vi "Copy Channel Information.vi"(8 "error in (no error)":errorcluster, 10 "new tdms file":refnum<k34>, 11 "original tdms file":refnum<k34>) -> (0 "error out":errorcluster, 3 "dup original tdms file":refnum<k34>)   [LabVIEW 2023]
doc: "Get all the meta information from the original file and dump them to the new file with TDMS Set Channel Information."
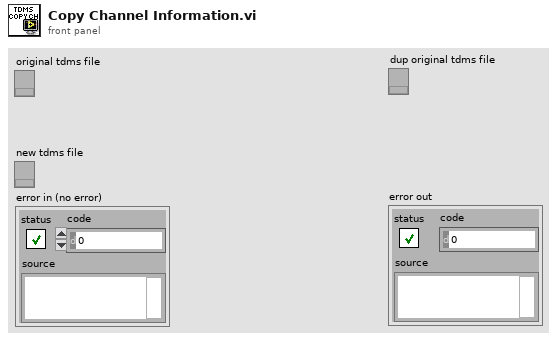
[diagram p1: front panel]
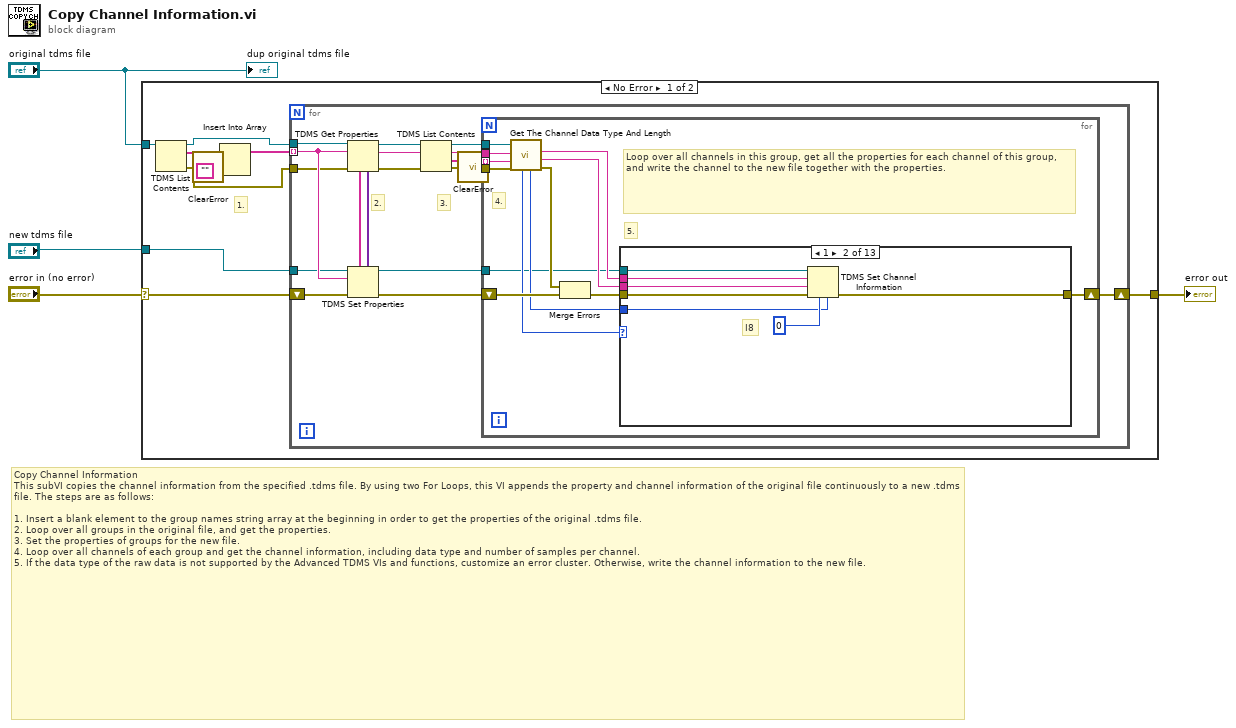
[diagram p0: block diagram]
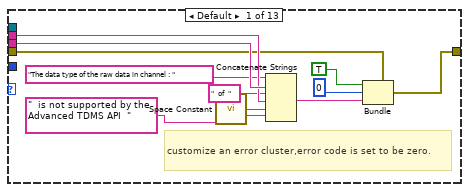
[diagram p2: hidden frame]
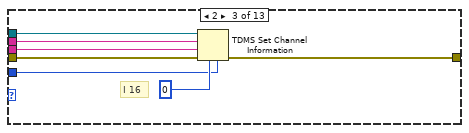
[diagram p3: hidden frame]
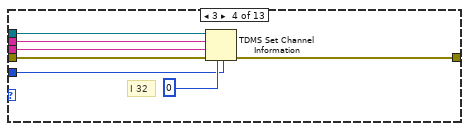
[diagram p4: hidden frame]
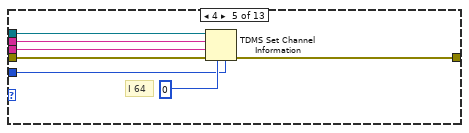
[diagram p5: hidden frame]
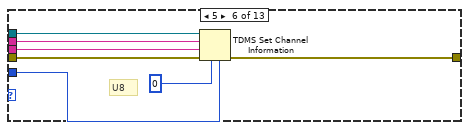
[diagram p6: hidden frame]
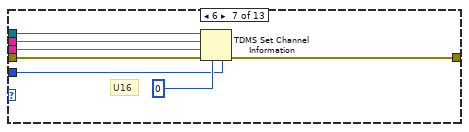
[diagram p7: hidden frame]
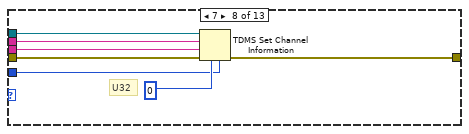
[diagram p8: hidden frame]
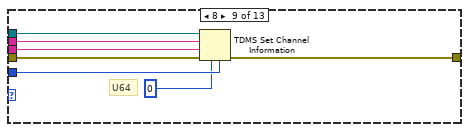
[diagram p9: hidden frame]
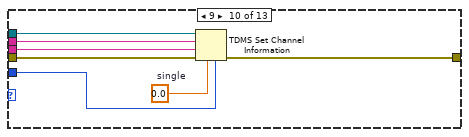
[diagram p10: hidden frame]
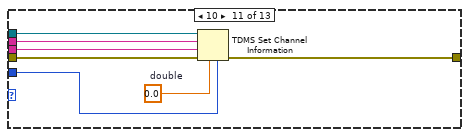
[diagram p11: hidden frame]
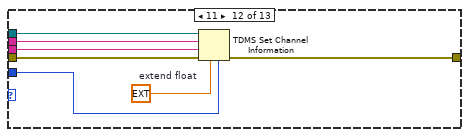
[diagram p12: hidden frame]
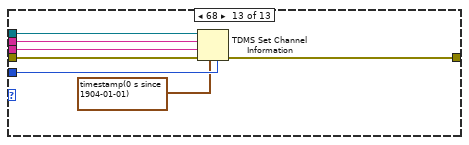
[diagram p13: hidden frame]
diagram:
  # "Copy Channel Information\nThis subVI copies the channel information from the specified .tdms file. By using two For Loops, this VI appends the property and channel information of the original file continuously to a new .tdms file. The steps are as follows:\n\n1. Insert a blank element to the group names string array at the beginning in order to get the properties of the original .tdms file.\n2. Loop over all groups in the original file, and get the properties.\n3. Set the properties of groups for the new file.\n4. Loop over all channels of each group and get the channel information, including data type and number of samples per channel.\n5. If the data type of the raw data is not supported by the Advanced TDMS VIs and functions, customize an error cluster. Otherwise, write the channel information to the new file."
  n1 = case shown="No Error" "error in (no error)" {
    selector: "error in (no error)" -> [w8 w141]
    tunnel: "new tdms file" -> [w6 _]
    tunnel: [w14 w141] -> w3
    tunnel: "original tdms file" -> [w11 _]
    frame No Error {
      # "1."
      n2 = TDMS List Contents(7:w11) -> (0:w5:errorcluster, 2:w9:string[], 3:w10:refnum<k34>)  [unwired: 2 in, 1 out]
      n3 = call <vilib>:"ClearError.vi"("error in (no error)"=w5) -> ("error out"=w7:errorcluster)
      n4 = Insert Into Array(array=w9, new element="" ("new element/subarray")) -> (w12:string[])  [unwired: 1 in]
      n5 = for {
        tunnel: w12 -> [w20] mode=indexing
        shift-right: [w29] -> w14
        shift-left: w8 -> [w18]
        tunnel: w7 -> [w19]
        tunnel: w10 -> [w30]
        tunnel: w6 -> [w17]
        # "3."
        # "2."
        n6 = TDMS Get Properties(8:w19, 10:w20, 11:w30) -> (0:w23:errorcluster, 2:w27:string, 3:w28:refnum<k34>, 4:w31:variant[], 6:w32:string[])  [unwired: 3 in, 1 out]
        n7 = TDMS Set Properties(5:w31, 7:w32, 8:w18, 10:w20, 11:w17) -> (0:w21:errorcluster, 3:w16:refnum<k34>)  [unwired: 1 in, 2 out]
        n8 = TDMS List Contents(4:w23, 6:w27, 7:w28) -> (0:w15:errorcluster, 1:w24:string[], 2:w25:string, 3:w26:refnum<k34>)
        n9 = call <vilib>:"ClearError.vi"("error in (no error)"=w15) -> ("error out"=w22:errorcluster)
        n10 = for {
          shift-right: [w45] -> w29
          shift-left: w21 -> [w38]
          tunnel: w25 -> [w41]
          tunnel: w24 -> [w40] mode=indexing
          tunnel: w22 -> [w39]
          tunnel: w26 -> [w42]
          tunnel: w16 -> [w33]
          # "5."
          # "4."
          # "Loop over all channels in this group, get all the properties for each channel of this group, and write the channel to the new file together with the properties."
          n11 = call "Get The Channel Data Type And Length.vi"("error in (no error)"=w39, "channel name"=w40, "group name"=w41, "tdms file"=w42) -> ("error out"=w44:errorcluster, "dup channel name"=w34:string, "dup group name"=w35:string, "channel length"=w37:i32, "data type"=w36:i32)  [unwired: 2 in, 1 out]
          n12 = Merge Errors(w44, w38) -> (w43:errorcluster)
          n13 = case shown="1" w36 {
            tunnel: w37 -> [_ w62 w68 w76 w83 w85 w96 w103 w112 w113 w120 w127 w139]
            tunnel: w33 -> [_ w61 w70 w75 w82 w91 w98 w105 w110 w118 w125 w133 w140]
            tunnel: w35 -> [w54 w60 w66 w74 w81 w90 w95 w102 w109 w117 w123 w131 w137]
            tunnel: w34 -> [w56 w59 w67 w73 w80 w89 w94 w101 w108 w116 w124 w132 w136]
            tunnel: w43 -> [w50 w58 w65 w72 w79 w87 w93 w100 w107 w115 w122 w130 w135]
            tunnel: [w46 w57 w64 w71 w78 w86 w92 w99 w106 w114 w121 w129 w134] -> w45
            frame Default {
              # "customize an error cluster,error code is set to be zero."
              n14 = call <vilib>:"Space Constant.vi"() -> ("String"=w55:string)
              n15 = Concatenate Strings("The data type of the raw data in channel : " ("message"), w56, "  of  ", w54, w55, "  is not supported by the Advanced TDMS API  " ("message")) -> (w49:string)
              n16 = Bundle(cluster=w50, "status"=TRUE, "code"=0, "source"=w49) -> (w46:errorcluster)
            }
            frame 1 {
              # "I8"
              n17 = TDMS Set Channel Information(4:w62, 6:i8 0, 8:w58, 9:w59, 10:w60, 11:w61) -> (0:w57:errorcluster)  [unwired: 1 in, 1 out]
            }
            frame 2 {
              # "I 16"
              n18 = TDMS Set Channel Information(4:w68, 6:i16 0, 8:w65, 9:w67, 10:w66, 11:w70) -> (0:w64:errorcluster)  [unwired: 1 in, 1 out]
            }
            frame 3 {
              # "I 32"
              n19 = TDMS Set Channel Information(4:w76, 6:0, 8:w72, 9:w73, 10:w74, 11:w75) -> (0:w71:errorcluster)  [unwired: 1 in, 1 out]
            }
            frame 4 {
              # "I 64"
              n20 = TDMS Set Channel Information(4:w83, 6:i64 0, 8:w79, 9:w80, 10:w81, 11:w82) -> (0:w78:errorcluster)  [unwired: 1 in, 1 out]
            }
            frame 5 {
              # "U8"
              n21 = TDMS Set Channel Information(4:w85, 6:u8 0, 8:w87, 9:w89, 10:w90, 11:w91) -> (0:w86:errorcluster)  [unwired: 1 in, 1 out]
            }
            frame 6 {
              # "U16"
              n22 = TDMS Set Channel Information(4:w96, 6:u16 0, 8:w93, 9:w94, 10:w95, 11:w98) -> (0:w92:errorcluster)  [unwired: 1 in, 1 out]
            }
            frame 7 {
              # "U32"
              n23 = TDMS Set Channel Information(4:w103, 6:u32 0, 8:w100, 9:w101, 10:w102, 11:w105) -> (0:w99:errorcluster)  [unwired: 1 in, 1 out]
            }
            frame 8 {
              # "U64"
              n24 = TDMS Set Channel Information(4:w112, 6:u64 0, 8:w107, 9:w108, 10:w109, 11:w110) -> (0:w106:errorcluster)  [unwired: 1 in, 1 out]
            }
            frame 9 {
              w119 = sgl 0.0  # single
              n25 = TDMS Set Channel Information(4:w113, 6:w119, 8:w115, 9:w116, 10:w117, 11:w118) -> (0:w114:errorcluster)  [unwired: 1 in, 1 out]
            }
            frame 10 {
              w126 = 0.0  # double
              n26 = TDMS Set Channel Information(4:w120, 6:w126, 8:w122, 9:w124, 10:w123, 11:w125) -> (0:w121:errorcluster)  [unwired: 1 in, 1 out]
            }
            frame 11 {
              w128 = ext 0.0  # extend float
              n27 = TDMS Set Channel Information(4:w127, 6:w128, 8:w130, 9:w132, 10:w131, 11:w133) -> (0:w129:errorcluster)  [unwired: 1 in, 1 out]
            }
            frame 68 {
              n28 = TDMS Set Channel Information(4:w139, 6:timestamp(0 s since 1904-01-01), 8:w135, 9:w136, 10:w137, 11:w140) -> (0:w134:errorcluster)  [unwired: 1 in, 1 out]
            }
          }
        }
      }
    }
    frame Error {
    }
  }
  "error out" <- w3
  "dup original tdms file" <- "original tdms file"
